vi "Read Write.vi"(8 "error in (no error)":errorcluster, 10 "Write String":string, 11 "VISA resource name":refnum<visa-resource-name>) -> (0 "error out":errorcluster, 2 "Read Data":string, 3 "VISA resource name out":refnum<visa-resource-name>)   [LabVIEW 2015, in "Fluke 8808.lvlib"]
doc: "Issues commands and reads responses from the instrument."
uses:
  <instrlib>/Fluke 8808/Fluke 8808.lvlib
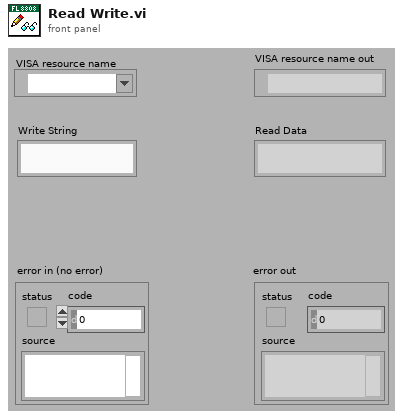
[diagram p1: front panel]
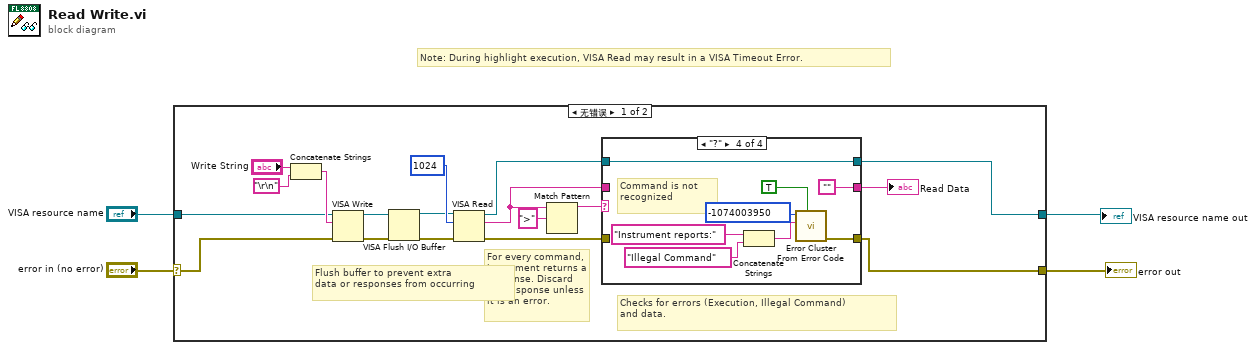
[diagram p0: block diagram]
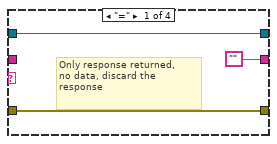
[diagram p2: hidden frame]
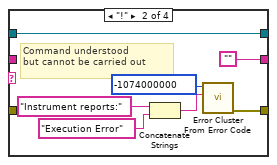
[diagram p3: hidden frame]
diagram:
  # "Note: During highlight execution, VISA Read may result in a VISA Timeout Error."
  n1 = case shown="无错误" "error in (no error)" {
    selector: "error in (no error)" -> [w5 w45]
    tunnel: "VISA resource name" -> [w13 w44]
    tunnel: [w7 w45] -> w2
    tunnel: [w6 w44] -> w1
    frame No Error {
      # "Flush buffer to prevent extra\ndata or responses from occurring"
      # "Checks for errors (Execution, Illegal Command)\nand data."
      # "For every command, instrument returns a response. Discard the response unless it is an error."
      n2 = Concatenate Strings("Write String", "\r\n") -> (w22:string)
      n3 = VISA Write(VISA resource name=w13, write buffer=w22, error in (no error)=w5) -> (VISA resource name out=w12:refnum<visa-resource-name>, error out=w11:errorcluster)  [unwired: 1 out]
      n4 = VISA Flush I/O Buffer(VISA resource name=w12, error in (no error)=w11) -> (VISA resource name out=w10:refnum<visa-resource-name>, error out=w9:errorcluster)  [unwired: 1 in]
      n5 = VISA Read(VISA resource name=w10, byte count=u32 1024, error in (no error)=w9) -> (VISA resource name out=w8:refnum<visa-resource-name>, read buffer=w16:string, error out=w15:errorcluster)  [unwired: 1 out]
      n6 = Match Pattern(string=w16, regular expression=">") -> (before substring=w18:string)  [unwired: 1 in, 3 out]
      n7 = case shown="\"?\"" w18 {
        tunnel: w16 -> [_ _ w33 _]
        tunnel: w15 -> [w25 _ w35 _]
        tunnel: [w25 w31 w35 w40] -> w7
        tunnel: ["" "" w33 ""] -> w14
        tunnel: w8 -> [w24 w27 w34 w37]
        tunnel: [w24 w27 w34 w37] -> w6
        frame "=" {
          # "Only response returned,\nno data, discard the \nresponse"
        }
        frame "!" {
          # "Command understood\nbut cannot be carried out"
          n8 = Concatenate Strings("Instrument reports:" ("Source"), "Execution Error" ("read buffer")) -> (w28:string)
          n9 = call <vilib>:"Error Cluster From Error Code.vi"("error message (\"\")"=w28, "error code (0)"=-1074000000 ("Code")) -> ("error out"=w31:errorcluster)  [unwired: 7 in]
        }
        frame Default {
          # "Returns data immediately"
        }
        frame "?" {
          # "Command is not\nrecognized"
          n10 = Concatenate Strings("Instrument reports:" ("Source"), "Illegal Command" ("read buffer")) -> (w41:string)
          n11 = call <vilib>:"Error Cluster From Error Code.vi"("show call chain? (False)"=TRUE, "error message (\"\")"=w41, "error code (0)"=-1074003950 ("Code")) -> ("error out"=w40:errorcluster)  [unwired: 6 in]
        }
      }
      "Read Data" <- w14
    }
    frame Error {
    }
  }
  "VISA resource name out" <- w1
  "error out" <- w2
